vi "Get Sequence Call Step Reference.vi"(8 "error in (no error)":errorcluster, 10 "Sequence Call to Retrieve":string, 11 "Sequence Call Step Dict in":refnum<class "Sequence Call Step Dictionary.lvclass">) -> (0 "error out":errorcluster, 2 "Sequence Call Step Out":T1, 3 "Sequence Call Step Dict out":refnum<class "Sequence Call Step Dictionary.lvclass">)   [LabVIEW 2018, in "Sequence Call Step Dictionary.lvlib" / "Sequence Call Step Dictionary.lvclass"]
doc: "Retrieves and clones Sequence Call Step"
uses:
  Sequence Call Step Dictionary.lvclass
  Controls/Sequence Call Step.ctl
  Controls/Parameter.ctl
  Sequence Call Step Dictionary.lvclass/Sequence Call Step Dictionary.ctl
  Private Methods/Read Database.vi
  <vilib>/ErrorRing/Error Ring.xnode
  Plugins/TestStand API Tools (TSAT).lvlibp/Step Actions/TSAT Step Actions.lvlib
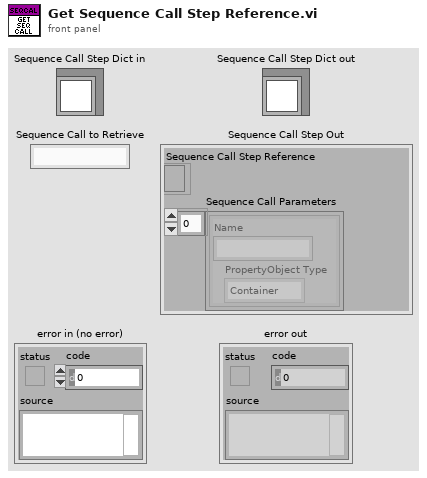
[diagram p1: front panel]
types:
  T1 = typedef "Sequence Call Step Dictionary.lvlib/Sequence Call Step Dictionary.lvclass/Sequence Call Step.ctl" = cluster{"Sequence Call Step Reference":refnum<k7>, "Sequence Call Parameters":T2[]}
  T2 = typedef "Sequence Call Step Dictionary.lvlib/Sequence Call Step Dictionary.lvclass/Parameter.ctl" = cluster{"Name":string, "PropertyObject Type":enum16{"Container", "String", "Boolean", "Number", "NamedType", "Reference", "Array", "Aperture Time"}}
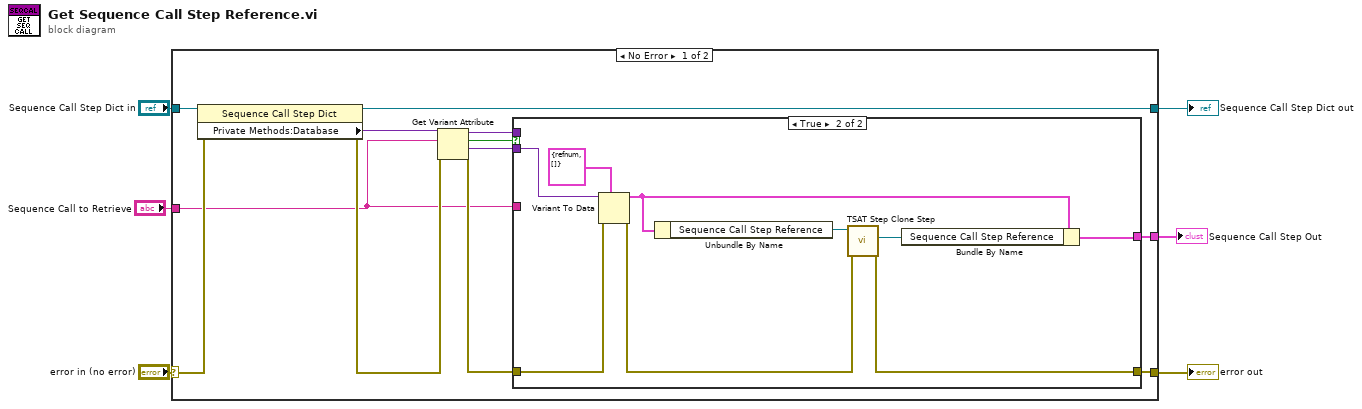
[diagram p0: block diagram]
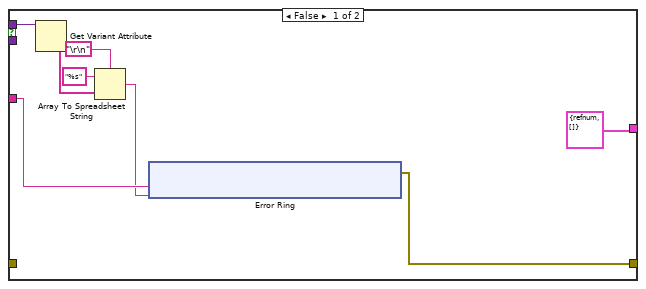
[diagram p2: hidden frame]
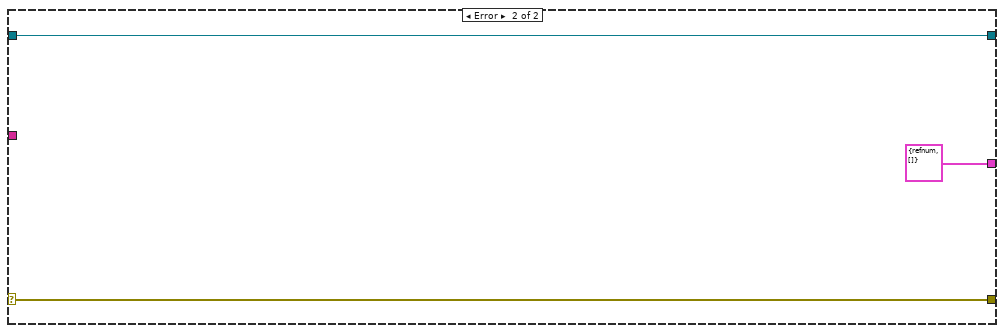
[diagram p3: hidden frame]
diagram:
  n1 = case shown="No Error" "error in (no error)" {
    selector: "error in (no error)" -> [w18 w44]
    tunnel: [w11 w44] -> w5
    tunnel: [w16 w43] -> w3
    tunnel: "Sequence Call Step Dict in" -> [w17 w43]
    tunnel: "Sequence Call to Retrieve" -> [w7 _]
    tunnel: [w8 T1 {"Sequence Call Step Reference"=refnum, "Sequence Call Parameters"=[]} ("Cluster")] -> w1
    frame No Error {
      n2 = property class="Sequence Call Step Dict"(reference=w17, error in=w18) -> (reference out=w16:refnum<class "Sequence Call Step Dictionary.lvclass">, error out=w14:errorcluster, "Private Methods:Database"=w15:variant)
      n3 = Get Variant Attribute(Variant=w15, name=w7, error in=w14) -> (duplicate Variant=w9:variant, found=w10:bool, value=w13:variant, error out=w12:errorcluster)  [unwired: 1 in]
      n4 = case shown="True" w10 {
        tunnel: w13 -> [_ w41]
        tunnel: w12 -> [_ w40]
        tunnel: [w23 w36] -> w11
        tunnel: w9 -> [w24 _]
        tunnel: [T1 {"Sequence Call Step Reference"=refnum, "Sequence Call Parameters"=[]} ("Cluster") w33] -> w8
        tunnel: w7 -> [w25 _]
        frame False {
          n5 = Get Variant Attribute(Variant=w24) -> (names=w22:string[])  [unwired: 3 in, 3 out]
          n6 = Array To Spreadsheet String(delimiter (Tab)="\r\n", array=w22, 3:"%s" ("format string")) -> (spreadsheet string=w19:string)
          n7 = xnode "Error Ring"("parameter 0"=w25, "parameter 1"=w19) -> ("error out"=w23:errorcluster)
        }
        frame True {
          n8 = Variant To Data(error in=w40, type=T1 {"Sequence Call Step Reference"=refnum, "Sequence Call Parameters"=[]} ("Cluster"), Variant=w41) -> (data=w35:T1, error out=w37:errorcluster)
          n9 = Unbundle By Name(w35) -> ("Sequence Call Step Reference"=w38:refnum<k7>)
          n10 = call "TSAT Step Clone Step.vi"("Error In"=w37, "Step In"=w38) -> ("Error Out"=w36:errorcluster, "Cloned Step"=w34:refnum<k7>)  [unwired: 7 in, 1 out]
          n11 = Bundle By Name(cluster=w35, "Sequence Call Step Reference"=w34) -> (w33:T1)
        }
      }
    }
    frame Error {
    }
  }
  "error out" <- w5
  "Sequence Call Step Dict out" <- w3
  "Sequence Call Step Out" <- w1
